vi "SRV.vi"() -> ()   [LabVIEW 2020]
panel:
  out "number":dbl
  out "offset past number":i32
  out "data out":string
  out "vit":dbl(knob) scale=-1.0..1.0
  in  "stop":bool
  in  "Port":u16
  out "error out":errorcluster
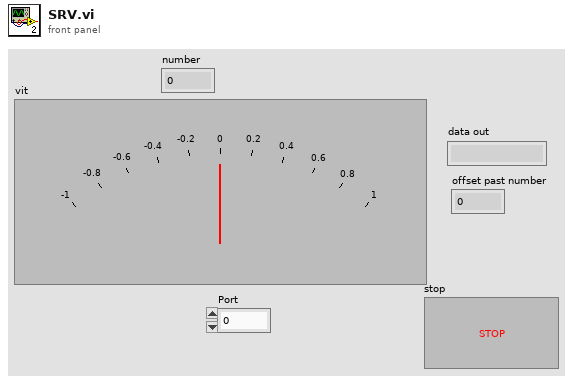
[diagram p1: front panel]
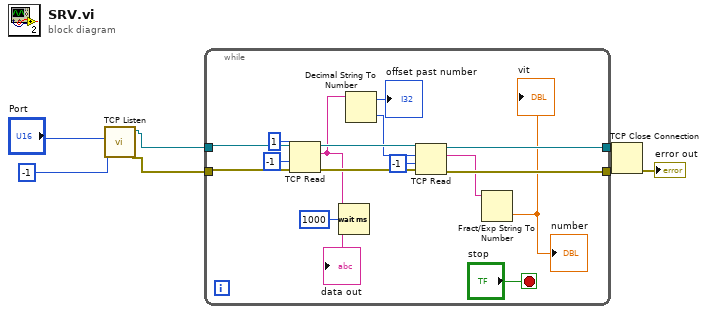
[diagram p0: block diagram]
diagram:
  n1 = call <vilib>:"TCP Listen.vi"("timeout ms (wait forever: -1)"=-1 ("timeout ms (60000)"), "port"="Port") -> ("error out"=w3:errorcluster, "connection ID"=w4:refnum<k5>)  [unwired: 5 in, 3 out]
  n2 = while {
    tunnel: w4 -> [w22]
    tunnel: [w20] -> w7
    tunnel: w3 -> [w19]
    tunnel: [w17] -> w6
    stop <- "stop" stop-if-true
    n3 = TCP Read(connection ID=w22, bytes to read=1, error in (no error)=w19, 9:-1 ("timeout ms (25000)")) -> (connection ID out=w21:refnum<k5>, data out=w14:string, error out=w18:errorcluster)  [unwired: 1 in]
    "data out" <- w14
    n4 = Wait (ms)(milliseconds to wait=u32 1000) -> ()  [unwired: 1 out]
    n5 = Decimal String To Number(string=w14) -> (offset past number=→"offset past number":i32, number=w13:i32)  [unwired: 2 in]
    n6 = TCP Read(connection ID=w21, bytes to read=w13, error in (no error)=w18, 9:-1 ("timeout ms (25000)")) -> (connection ID out=w20:refnum<k5>, data out=w16:string, error out=w17:errorcluster)  [unwired: 1 in]
    n7 = Fract/Exp String To Number(string=w16) -> (number=→"vit" →"number":dbl)  [unwired: 3 in, 1 out]
  }
  n8 = TCP Close Connection(connection ID=w7, error in (no error)=w6) -> (error out=→"error out":errorcluster)  [unwired: 1 in, 1 out]
